vi "Get PK Column.vi"(8 "error in (no error)":errorcluster, 11 "Table Configuration Interface in":refnum<class "Table Configuration Interface.lvclass">) -> (0 "error out":errorcluster, 2 "Primary Key":T1, 3 "Table Configuration Interface out":refnum<class "Table Configuration Interface.lvclass">)   [LabVIEW 2020, in "Table.lvlib" / "Table Configuration Interface.lvclass"]
uses:
  Table Configuration Interface.lvclass
  Database Libraries/Database Interfaces/Primary Key Info.ctl
  Database Libraries/Database Interfaces.lvlib
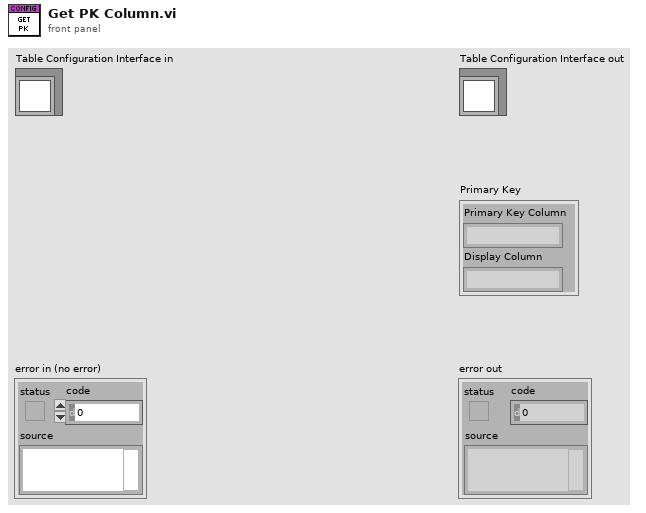
[diagram p1: front panel]
types:
  T1 = typedef "Database Interfaces.lvlib/Primary Key Info.ctl" = cluster{"Primary Key Column":string, "Display Column":string}
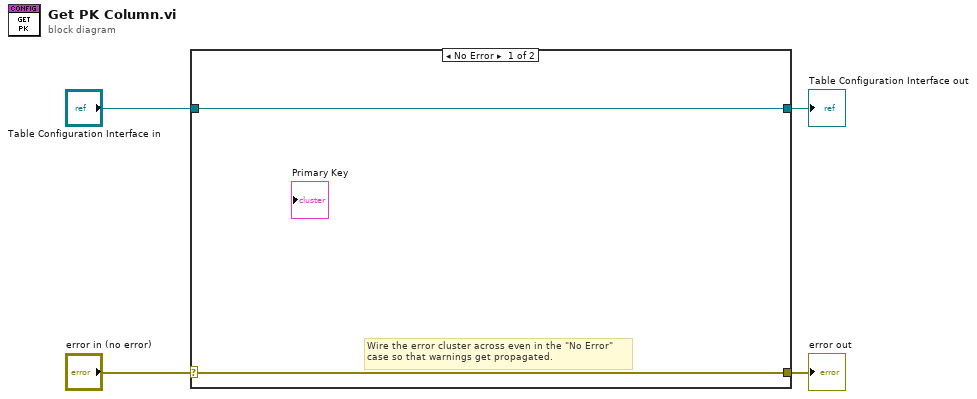
[diagram p0: block diagram]
diagram:
  n1 = case shown="No Error" "error in (no error)" {
    selector: "error in (no error)" -> [w5 w8]
    tunnel: [w5 w8] -> w3
    tunnel: [w6 w7] -> w1
    tunnel: "Table Configuration Interface in" -> [w6 w7]
    frame No Error {
      # "Wire the error cluster across even in the \"No Error\"\ncase so that warnings get propagated."
    }
    frame Error {
    }
  }
  "error out" <- w3
  "Table Configuration Interface out" <- w1
